vi "ArraySample.vi"() -> ()   [LabVIEW 2025]
doc: "Iterates through numeric, boolean, and string arrays using a For Loop to update each element with a modified value."
panel:
  out "Updated boolean array":bool[](array[boolean])
  out "Updated numeric array":dbl[](array[numeric])
  in  "Array 7":string[](array[string])
  in  "Boolean array":bool[](array[boolean])
  in  "Numeric array":dbl[](array[numeric])
  # "Working with numeric, boolean,string arrays inside for loop by updating each value in array"
  # "string array for length"
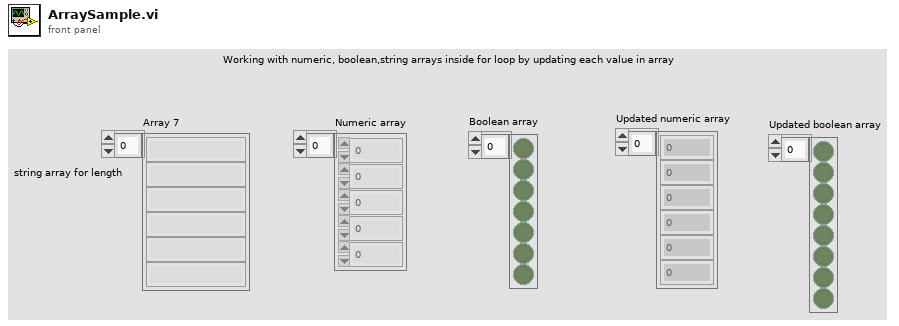
[diagram p1: front panel]
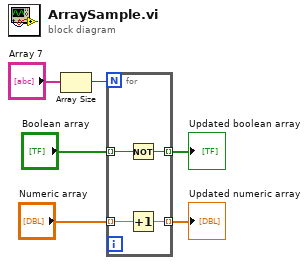
[diagram p0: block diagram]
diagram:
  n1 = Array Size(array="Array 7") -> (size(s)=w5:i32)
  n2 = for {
    N: w5 -> [_]
    tunnel: "Numeric array" -> [w10] mode=indexing
    tunnel: [w9] -> w3 mode=indexing
    tunnel: "Boolean array" -> [w8] mode=indexing
    tunnel: [w7] -> w1 mode=indexing
    n3 = Not(x=w8) -> (.not. x?=w7:bool)
    n4 = Increment(x=w10) -> (x+1=w9:dbl)
  }
  "Updated numeric array" <- w3
  "Updated boolean array" <- w1
